vi "TelemetryFieldToAddress.vi"(11 "TelemetryFields":T1) -> (3 "Address":u32)   [LabVIEW 2016]
uses:
  TelemetryFields.ctl
  <vilib>/Platform/TimedLoop/XDataNode/timing_clust.ctl
  <vilib>/Platform/TimedLoop/XDataNode/nitl_modes.ctl
  <vilib>/Platform/TimedLoop/XDataNode/wakeup.ctl
  <vilib>/rvi/Emulation/niFpgaSctlEmulationGetInTimedLoop.vi
  <vilib>/rvi/Emulation/niFpgaEmulationReportErrorSimple.vi
  <vilib>/rvi/Emulation/niFpgaGetClockAttributes.vi
  <vilib>/rvi/Emulation/niFpgaCriticalErrorInLSC.vi
  <vilib>/Platform/TimedLoop/XDataNode/XDataNode.xnode
  <vilib>/Platform/TimedLoop/XDataNode/XDNodeRunTimeDep.lvlib
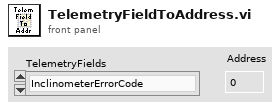
[diagram p1: front panel]
types:
  T1 = typedef "TelemetryFields.ctl" = enum16{"InclinometerErrorCode", "InclinometerTxBytes", "InclinometerRxBytes", "InclinometerTxFrames", "InclinometerRxFrames", "InclinometerTimestamp", "InclinometerAngle", "DisplacementErrorCode", "DisplacementTxBytes", "DisplacementRxBytes", "DisplacementTxFrames", "DisplacementRxFrames", "DisplacementTimestamp", "Displacement1", "Displacement2", "Displacement3", "Displacement4", "Displacement5", "Displacement6", "Displacement7", "Displacement8", "AccelerometerSampleCount", "AccelerometerTimestamp", "AccelerometerRaw1", "AccelerometerRaw2", "AccelerometerRaw3", "AccelerometerRaw4", "AccelerometerRaw5", "AccelerometerRaw6", "AccelerometerRaw7", "AccelerometerRaw8", "AccelerometerEng1", "AccelerometerEng2", "AccelerometerEng3", "AccelerometerEng4", "AccelerometerEng5", "AccelerometerEng6", "AccelerometerEng7", "AccelerometerEng8", "AngularAccelerationX", "AngularAccelerationY", "AngularAccelerationZ"}
  T2 = typedef "XDNodeRunTimeDep.lvlib/timing_clust.ctl" = cluster{"Expected End [f-1]":u64, "Actual End [f-1]":u64, "Finished Late? [f-1]":bool, "Expected End [i-1]":u64, "Actual End [i-1]":u64, "Finished Late? [i-1]":bool, "Expected Start [i]":u64, "Actual Start [i]":u64, "Expected Start [f]":u64, "Actual Start [f]":u64, "Source Name":string, "Structure Name":string, "Period":i64, "Deadline":i64, "Offset":i64, "Start":i64, "Priority":i32, "Timeout":i32, "Mode":T3, "Wakeup Reason":T4, "Error":errorcluster, "Source Type":string, "Secondary Source Type":string, "Global End Time":u64, "Global Start Time":u64, "Frame Duration":u64, "Iteration Duration":u64, "Assigned CPU":i32, "I/O Scan Engine Mode":u32}
  T3 = typedef "XDNodeRunTimeDep.lvlib/nitl_modes.ctl" = enum32{"No Change", "Process missed periods, maintain original phase", "Discard missed periods, maintain original phase", "Process missed periods, ignore original phase", "Discard missed periods, ignore original phase"}
  T4 = typedef "XDNodeRunTimeDep.lvlib/wakeup.ctl" = enum32{"Normal", "Aborted", "Asynchronous wakeup", "Timing source error", "Timed loop error", "Timeout"}
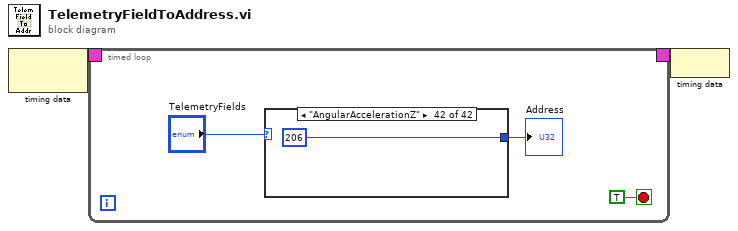
[diagram p0: block diagram]
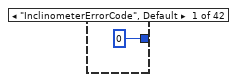
[diagram p2: hidden frame]
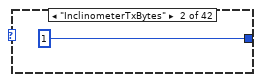
[diagram p3: hidden frame]
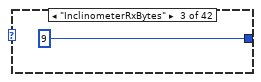
[diagram p4: hidden frame]
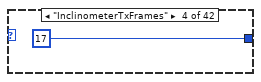
[diagram p5: hidden frame]
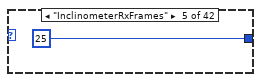
[diagram p6: hidden frame]
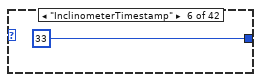
[diagram p7: hidden frame]
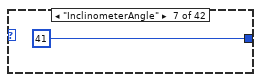
[diagram p8: hidden frame]
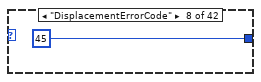
[diagram p9: hidden frame]
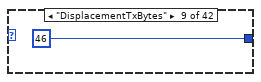
[diagram p10: hidden frame]
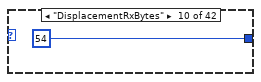
[diagram p11: hidden frame]
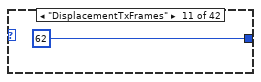
[diagram p12: hidden frame]
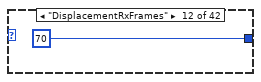
[diagram p13: hidden frame]
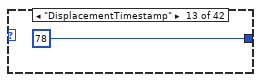
[diagram p14: hidden frame]
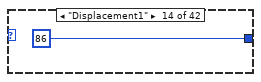
[diagram p15: hidden frame]
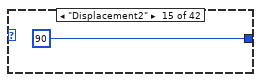
[diagram p16: hidden frame]
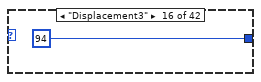
[diagram p17: hidden frame]
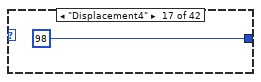
[diagram p18: hidden frame]
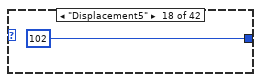
[diagram p19: hidden frame]
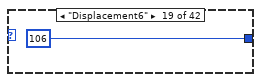
[diagram p20: hidden frame]
diagram:
  n1 = node-c288() -> (w2:T2)  [unwired: 1 in]
  n2 = timed-loop {
    timing: w2 -> [_]
    timing-out: [_] -> w1
    stop <- TRUE stop-if-true
    n3 = case shown="\"AngularAccelerationZ\"" "TelemetryFields" {
      tunnel: [u32 0 ("Address") u32 1 ("Address") u32 9 ("Address") u32 17 ("Address") u32 25 ("Address") u32 33 ("Address") u32 41 ("Address") u32 45 ("Address") u32 46 ("Address") u32 54 ("Address") u32 62 ("Address") u32 70 ("Address") u32 78 ("Address") u32 86 ("Address") u32 90 ("Address") u32 94 ("Address") u32 98 ("Address") u32 102 ("Address") u32 106 ("Address") u32 110 ("Address") u32 114 ("Address") u32 118 ("Address") u32 126 ("Address") u32 134 ("Address") u32 138 ("Address") u32 142 ("Address") u32 146 ("Address") u32 150 ("Address") u32 154 ("Address") u32 158 ("Address") u32 162 ("Address") u32 166 ("Address") u32 170 ("Address") u32 174 ("Address") u32 178 ("Address") u32 182 ("Address") u32 186 ("Address") u32 190 ("Address") u32 194 ("Address") u32 198 ("Address") u32 202 ("Address") u32 206 ("Address")] -> w3
      frame "InclinometerErrorCode", Default {
      }
      frame "InclinometerTxBytes" {
      }
      frame "InclinometerRxBytes" {
      }
      frame "InclinometerTxFrames" {
      }
      frame "InclinometerRxFrames" {
      }
      frame "InclinometerTimestamp" {
      }
      frame "InclinometerAngle" {
      }
      frame "DisplacementErrorCode" {
      }
      frame "DisplacementTxBytes" {
      }
      frame "DisplacementRxBytes" {
      }
      frame "DisplacementTxFrames" {
      }
      frame "DisplacementRxFrames" {
      }
      frame "DisplacementTimestamp" {
      }
      frame "Displacement1" {
      }
      frame "Displacement2" {
      }
      frame "Displacement3" {
      }
      frame "Displacement4" {
      }
      frame "Displacement5" {
      }
      frame "Displacement6" {
      }
      frame "Displacement7" {
      }
      frame "Displacement8" {
      }
      frame "AccelerometerSampleCount" {
      }
      frame "AccelerometerTimestamp" {
      }
      frame "AccelerometerRaw1" {
      }
      frame "AccelerometerRaw2" {
      }
      frame "AccelerometerRaw3" {
      }
      frame "AccelerometerRaw4" {
      }
      frame "AccelerometerRaw5" {
      }
      frame "AccelerometerRaw6" {
      }
      frame "AccelerometerRaw7" {
      }
      frame "AccelerometerRaw8" {
      }
      frame "AccelerometerEng1" {
      }
      frame "AccelerometerEng2" {
      }
      frame "AccelerometerEng3" {
      }
      frame "AccelerometerEng4" {
      }
      frame "AccelerometerEng5" {
      }
      frame "AccelerometerEng6" {
      }
      frame "AccelerometerEng7" {
      }
      frame "AccelerometerEng8" {
      }
      frame "AngularAccelerationX" {
      }
      frame "AngularAccelerationY" {
      }
      frame "AngularAccelerationZ" {
      }
    }
    "Address" <- w3
  }
  n4 = node-c288(w1) -> ()
